vi "meta_writeColumnBlock.vi"(8 "error in (no error)":errorcluster, 10 "meta_ColumnInfo":T1, 11 "meta file in":T4) -> (0 "error out":errorcluster, 3 "meta file out":T4)   [LabVIEW 2017, in "NI_ExcelFile.lvlib"]
uses:
  <vilib>/express/express shared/NI_ExcelFile/NI_ExcelFile.lvlib
  <vilib>/express/express shared/NI_ExcelFile/Ctrls/meta_file.ctl
  <vilib>/express/express shared/NI_ExcelFile/Ctrls/meta_Block.ctl
  <vilib>/express/express shared/NI_ExcelFile/Ctrls/meta_BlockType.ctl
  <vilib>/express/express shared/NI_ExcelFile/Ctrls/meta_ColumnInfo.ctl
  <vilib>/express/express shared/NI_ExcelFile/Ctrls/meta_ColumnInfo_2013.ctl
  <vilib>/express/express shared/NI_ExcelFile/Ctrls/DataType.ctl
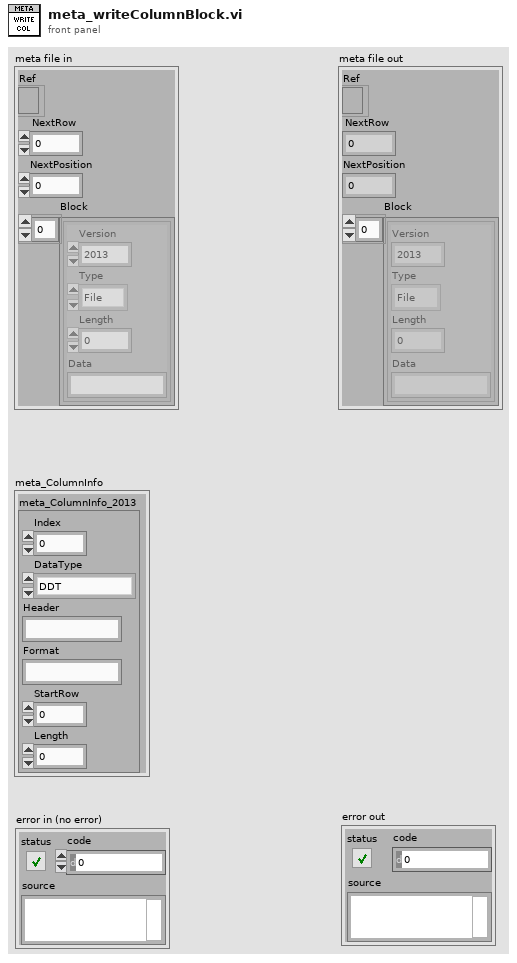
[diagram p1: front panel]
types:
  T1 = typedef "NI_ExcelFile.lvlib/meta_ColumnInfo.ctl" = cluster{"meta_ColumnInfo_2013":T2}
  T2 = typedef "NI_ExcelFile.lvlib/meta_ColumnInfo_2013.ctl" = cluster{"Index":i32, "DataType":T3, "Header":string, "Format":string, "StartRow":i32, "Length":i32}
  T3 = typedef "NI_ExcelFile.lvlib/DataType.ctl" = enum16{"DDT", "WFM", "Array of STR", "Array of DBL", "Array of I8", "Array of I16", "Array of I32", "Array of I64", "Array of SGL", "Array of U8", "Array of U16", "Array of U32", "Array of U64", "Array of Time"}
  T4 = typedef "NI_ExcelFile.lvlib/meta_file.ctl" = cluster{"Ref":refnum<file>, "NextRow":i32, "NextPosition":i64, "Block":T5[]}
  T5 = typedef "NI_ExcelFile.lvlib/meta_Block.ctl" = cluster{"Version":u16, "Type":T6, "Length":i32, "Data":string}
  T6 = typedef "NI_ExcelFile.lvlib/meta_BlockType.ctl" = enum16{"NITag", "File", "Column"}
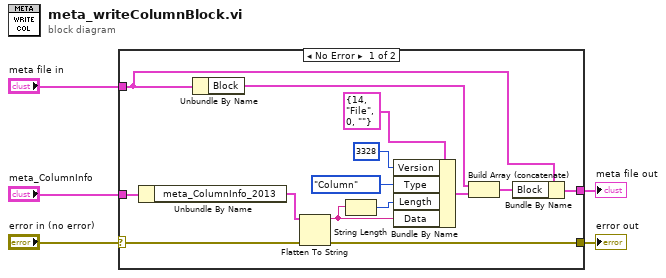
[diagram p0: block diagram]
diagram:
  n1 = case shown="No Error" "error in (no error)" {
    selector: "error in (no error)" -> [w12 w21]
    tunnel: "meta_ColumnInfo" -> [w18 _]
    tunnel: [w19 w20] -> w5
    tunnel: "meta file in" -> [w11 w20]
    tunnel: [w17 w21] -> w3
    frame No Error {
      n2 = Unbundle By Name(w18) -> ("meta_ColumnInfo_2013"=w14:T2)
      n3 = Unbundle By Name(w11) -> ("Block"=w16:T5[])
      n4 = Flatten To String(anything=w14, error in (no error)=w12) -> (data string=w13:string, error out=w17:errorcluster)  [unwired: 2 in, 1 out]
      n5 = String Length(string=w13) -> (length=w7:i32)
      n6 = Bundle By Name(cluster=T5 {"Version"=14, "Type"=enum."File", "Length"=0, "Data"=""} ("Block"), "Version"=u16 3328 ("version"), "Type"=meta_BlockType."Column" ("type"), "Length"=w7, "Data"=w13) -> (w6:T5)
      n7 = Build Array (concatenate)(w16, w6) -> (w15:T5[])
      n8 = Bundle By Name(cluster=w11, "Block"=w15) -> (w19:T4)
    }
    frame Error {
    }
  }
  "meta file out" <- w5
  "error out" <- w3
